vi "Test Trim Whitspace.vi"() -> ()   [LabVIEW 2017]
uses:
  JSONtext.lvlib
  <vilib>/Utility/error.llb/whitespace.ctl
  <userlib>/_OpenG.lib/string/string.llb/Trim Whitespace (String)__ogtk.vi
panel:
  in  "dimension size":i32=10
  out "x-y":dbl format="%#_6p"
  out "Array":string[](array[string])
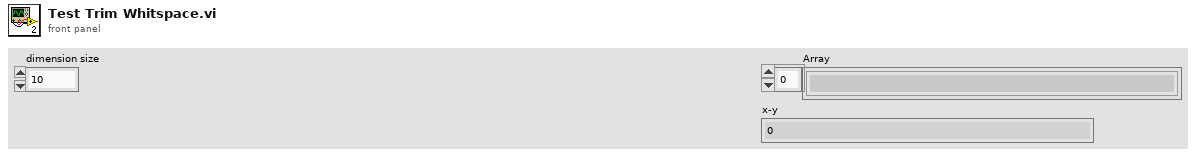
[diagram p1: front panel]
types:
  T1 = typedef "whitespace.ctl" = u16
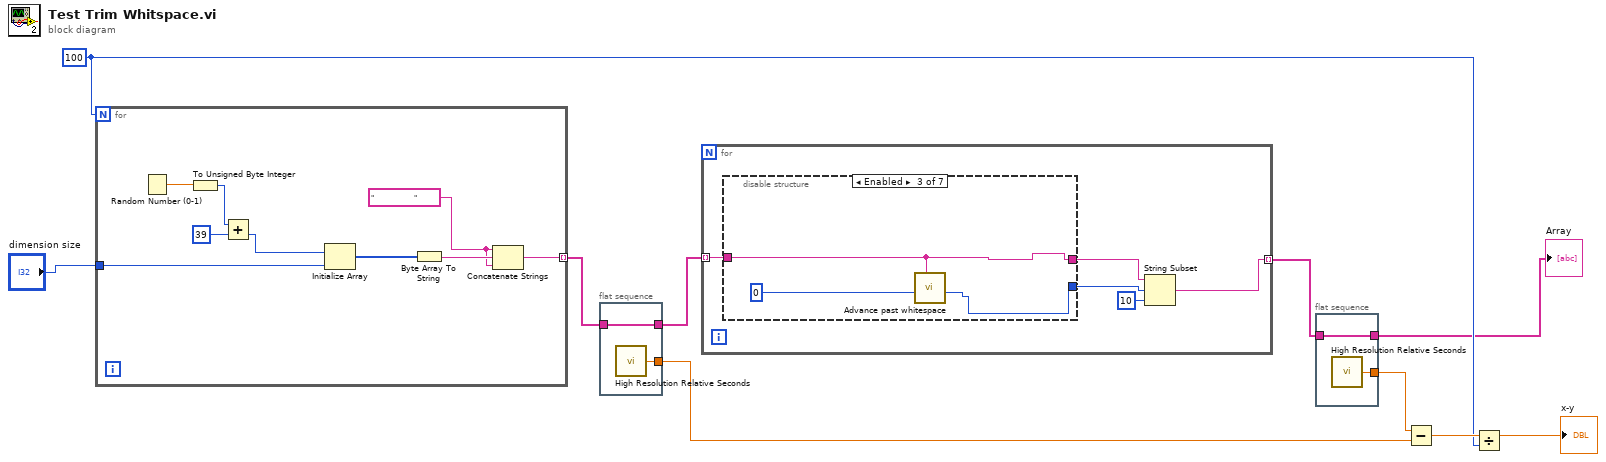
[diagram p0: block diagram]
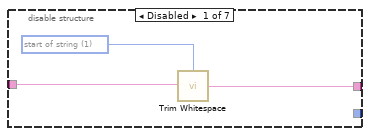
[diagram p2: hidden frame]
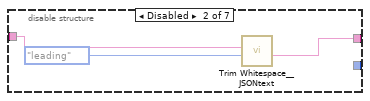
[diagram p3: hidden frame]
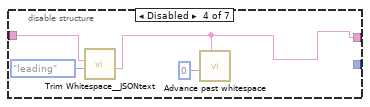
[diagram p4: hidden frame]
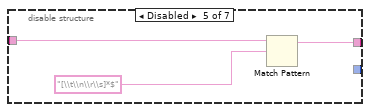
[diagram p5: hidden frame]
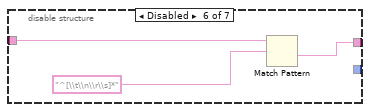
[diagram p6: hidden frame]
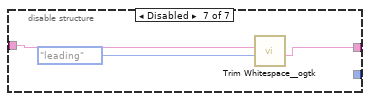
[diagram p7: hidden frame]
diagram:
  w2 = 100
  n1 = for {
    N: w2 -> [_]
    tunnel: [w15] -> w10 mode=indexing
    tunnel: "dimension size" -> [w11]
    w16 = "                    " ("element")
    n2 = Random Number (0-1)() -> (number: 0 to 1=w14:dbl)
    n3 = To Unsigned Byte Integer(number=w14) -> (unsigned 8bit integer=w12:u8)
    n4 = Add(x=w12, y=u8 39) -> (x+y=w13:u8)
    n5 = Initialize Array(w13, w11) -> (w18:u8[])
    n6 = Byte Array To String(unsigned byte array=w18) -> (string=w17:string)
    n7 = Concatenate Strings(w16, w17, w16) -> (w15:string)
  }
  n8 = flat-sequence {
    tunnel: [w21] -> w9
    tunnel: w10 -> [w21]
    tunnel: [w20] -> w6
    frame #0 {
      n9 = call <vilib>:"High Resolution Relative Seconds.vi"() -> ("relative seconds"=w20:dbl)
    }
  }
  n10 = for {
    tunnel: w9 -> [w26] mode=indexing
    tunnel: [w24] -> w8 mode=indexing
    n11 = disable-structure shown="Enabled" {
      disable-tunnel: w26 -> [w29 w32 w34 w38 w41 w44 w48]
      disable-tunnel: [w28 w31 w34 w36 w40 w43 w47] -> w25
      disable-tunnel: [_ _ w33 _ _ _ _] -> w22
      frame Disabled {
        w27 = T1 1 items=["both", "start of string", "end of string"] ("location (both)")
        n12 = call <vilib>:"Trim Whitespace.vi"("string"=w29, "location (both)"=w27) -> ("trimmed string"=w28:string)
      }
      frame Disabled {
        n13 = call "Trim Whitespace__JSONtext.vi"("Remove (leading and trailing)"=enum16{"leading", "trailing", "both"}."leading", "String in"=w32) -> ("String out"=w31:string)  [unwired: 5 in]
      }
      frame Enabled {
        n14 = call "Advance past whitespace.vi"("JSON"=w34, "Offset"=0) -> ("Offset of first non-whitespace"=w33:i32)  [unwired: 8 in, 1 out]
      }
      frame Disabled {
        n15 = call "Trim Whitespace__JSONtext.vi"("Remove (leading and trailing)"=enum16{"leading", "trailing", "both"}."leading", "String in"=w38) -> ("String out"=w36:string)  [unwired: 5 in]
        n16 = call "Advance past whitespace.vi"("JSON"=w36, "Offset"=0) -> ()  [unwired: 8 in, 2 out]
      }
      frame Disabled {
        n17 = Match Pattern(string=w41, regular expression="[\\t\\n\\r\\s]*$") -> (before substring=w40:string)  [unwired: 1 in, 3 out]
      }
      frame Disabled {
        n18 = Match Pattern(string=w44, regular expression="^[\\t\\n\\r\\s]*") -> (after substring=w43:string)  [unwired: 1 in, 3 out]
      }
      frame Disabled {
        n19 = call-poly <userlib>:"Trim Whitespace__ogtk.vi"("Remove (leading and trailing)"=enum16{"leading", "trailing", "both"}."leading", "String in"=w48) -> ("String out"=w47:string)  [unwired: 5 in]
      }
    }
    n20 = String Subset(string=w25, offset (0)=w22, length (rest)=10 ("length (rest)")) -> (substring=w24:string)
  }
  n21 = flat-sequence {
    tunnel: [w50] -> w1
    tunnel: w8 -> [w50]
    tunnel: [w49] -> w7
    frame #0 {
      n22 = call <vilib>:"High Resolution Relative Seconds.vi"() -> ("relative seconds"=w49:dbl)
    }
  }
  n23 = Subtract(x=w7, y=w6) -> (x-y=w5:dbl)
  n24 = Divide(x=w5, y=w2) -> (x/y=→"x-y":dbl)
  "Array" <- w1
